vi "Dashboard Main.vi"() -> ()   [LabVIEW 2020]
uses:
  <vilib>/Utility/miscctls.llb/LVRowAndColumnTypeDef.ctl
  <vilib>/event_ctls.llb/eventvkey.ctl
  <vilib>/Rock Robotics/Network Tables/NT Read Numeric Array.vi
  <vilib>/Rock Robotics/WPI/Dashboard/WPI_DashboardLogging Global.vi
panel:
  in  "Camera Settings Right":T1={"Frame Rate"=15, "Compression"=30, "Size"=1, "DB Camera Config"=FALSE} {"Frame Rate" scale=1.0..30.0; "Compression" scale=100.0..-1.0; "Size" items=["640x480", "320x240", "160x120"]}
  in  "Camera Name Right":string(combo)="No Camera Selection"
  out "Camera Perf":string="                          "
  in  "Camera Settings":T1={"Frame Rate"=15, "Compression"=30, "Size"=1, "DB Camera Config"=FALSE} {"Frame Rate" scale=1.0..30.0; "Compression" scale=100.0..-1.0; "Size" items=["640x480", "320x240", "160x120"]}
  in  "TCP":refnum<k5>
  in  "Rec Mode":enum32{"Stop", "Record", "Playback"}(radio)
  out "Robot IP":string="10.11.59.2"
  out "Image Message":string="Timeout in Camera Communications"
  in  "Dashboard Tab":T2(tab)=enum."Custom"
  in  "Select Pickup":string(combo)="Select Pickup ..."
  in  "Select Auto":string(combo)="Select Autonomous ..."
  out "NT Connection":bool
  out "MotorChart R":cluster{"Numeric":dbl, "Numeric":dbl}(graph)
  out "MotorChart L":cluster{"Numeric":dbl, "Numeric":dbl}(graph)
  out "MotorSliders R":cluster{"MotorSlide1":dbl, "MotorSlide2":dbl} {"MotorSlide2" scale=-1.0..1.0 scale format="%#_2e"; "MotorSlide1" scale=-1.0..1.0 scale format="%#_2e"}
  out "MotorSliders L":cluster{"MotorSlide1":dbl, "MotorSlide2":dbl} {"MotorSlide2" scale=-1.0..1.0 scale format="%#_2e"; "MotorSlide1" scale=-1.0..1.0 scale format="%#_2e"}
  out "Gyro":dbl(knob) scale=0.0..360.0
  out "JS1 Z":dbl(slide) scale=-1.0..1.0 scale format="%#_2e"
  out "JS1 Graph":cluster{"X":dbl, "Y":dbl}[](graph)
  out "JS1 Buttons":T3
  out "JS2 Z":dbl(slide) scale=-1.0..1.0 scale format="%#_2e"
  out "JS2 Graph":cluster{"X":dbl, "Y":dbl}[](graph)=[{"X"=0.0, "Y"=-0.007874015748031496}]
  out "JS2 Buttons":T3
  out "Mode":T4(ring)=enum."No Code"
  out "Right Camera Perf":cluster{"Bandwidth (Mbps)":dbl, "FPS":dbl}
  out "Camera Image Right":T5(plugin-control)
  in  "DB/String 9":string
  in  "DB/String 8":string
  in  "DB/String 7":string
  in  "DB/String 6":string
  in  "DB/String 5":string
  in  "DB/String 4":string
  in  "DB/String 3":string
  in  "DB/String 2":string
  in  "DB/String 1":string
  in  "DB/String 0":string
  in  "DB/Slider 0":dbl(slide) scale=0.0..5.0
  in  "DB/Slider 1":dbl(slide) scale=0.0..5.0
  in  "DB/Slider 2":dbl(slide) scale=0.0..5.0
  in  "DB/Slider 3":dbl(slide) scale=0.0..5.0
  out "DB/LED 3":bool
  out "DB/LED 2":bool
  out "DB/LED 1":bool
  out "DB/LED 0":bool
  in  "DB/Button 3":bool
  in  "DB/Button 2":bool
  in  "DB/Button 1":bool
  in  "DB/Button 0":bool caption="New Name"
  in  "Pivot Duration":dbl=1.0
  in  "Pivot Right Speed":dbl=-0.5
  in  "Pivot Left Speed":dbl=0.5
  in  "Transfer Release Duration":dbl=3.0
  in  "Transfer Up Duration":dbl=3.0
  in  "Intake Duration":dbl=5.0
  in  "Shooter Duration":dbl=3.0
  in  "Transfer Release Setpoint":dbl=1.0
  in  "Transfer Up Setpoint":dbl=1.0
  in  "Intake Setpoint":dbl=0.6
  in  "Shooter Setpoint":dbl=1.0
  in  "Test Slider":dbl(slide) scale=0.0..100.0 scale format="%#_3g"
  in  "On/Off":bool caption="Solenoid"
  in  "Test Name":u16(ring) items=["Select the test to run..."]
  in  "Test Tree":string(tree)
  in  "Motor":cluster{"Value":dbl, "Enable":bool} {"Value" scale=-1.0..1.0 scale format="%#_3g"}
  out "Progress":T6 {"Test Progress" scale=0.0..100.0}
  in  "Rev/Fwd":cluster{"Forward":bool, "Reverse":bool}
  in  "Test Ring":u16(ring) items=["Monochrome", "Color"]
  out "Cmd Status":string
  in  "Execute Command":bool
  in  "Command Params":string[][](table)
  in  "Command Selection":i32(listbox)
  in  "CheckList":i32(listbox)
  out "Tree":string(tree)
  out "Camera Image":T5(plugin-control)
  out "Background":bool
  in  "Camera Name":string(combo)="No Camera Selection"
  # "HW"
  # "HW"
  # "Joysticks"
  # "Drive Motors"
  # "Front"
  # "Right"
  # "Left"
  # "Back"
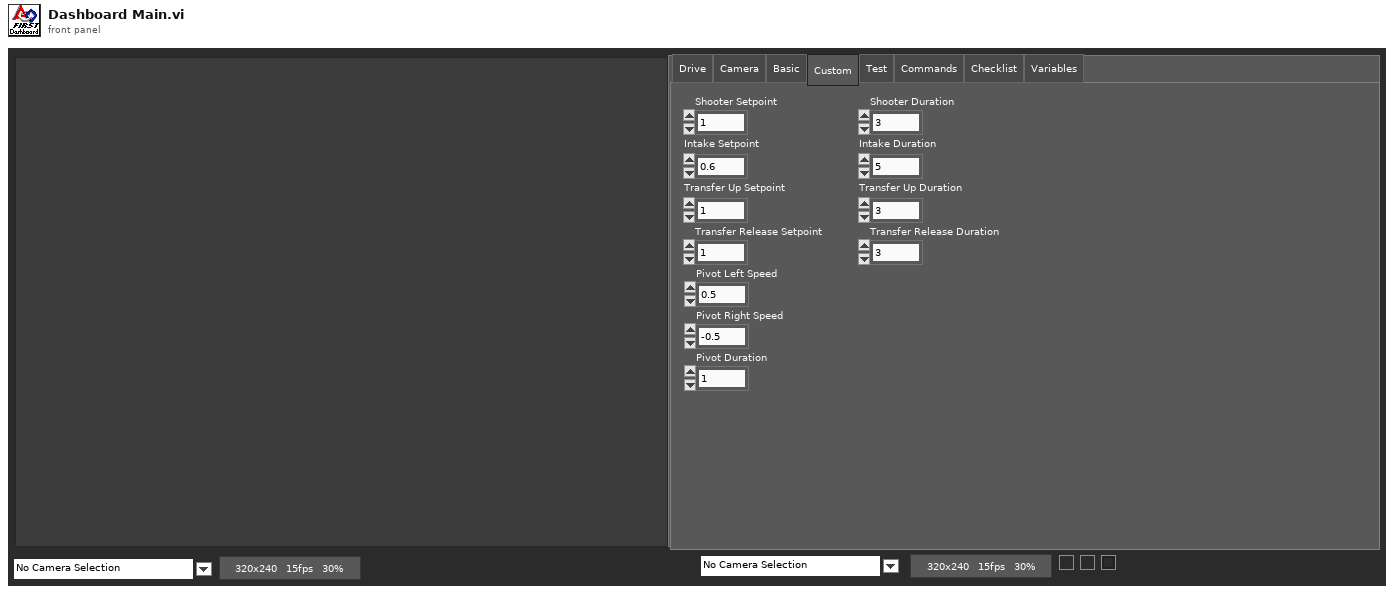
[diagram p1: front panel]
types:
  T1 = cluster{"Frame Rate":i32, "Compression":i32, "Size":u16, "DB Camera Config":bool}
  T2 = enum32{"Drive", "Camera", "Basic", "Custom", "Test", "Commands", "Checklist", "Variables"}
  T3 = cluster{bool, bool, bool, bool, bool, bool, bool, bool, bool, bool, bool, bool}
  T4 = enum8{"Tele-Op Disabled", "Tele-Op Enabled", "Auto Disabled", "Auto Enabled", "Test Disabled", "Test Enabled", "Disconnected", "No Code", "E-Stop"}
  T5 = typedef "IMAQ Image.ctl" = refnum<image>
  T6 = cluster{"Test Progress":u8, "Test Progress Text":string}
  T7 = cluster{"Save Path":path, "Interval (s)":dbl, "Keep":i32}
  T8 = typedef "Image Type" = u32
  T9 = cluster{"IDs":cluster{"RPC field ID":u16, "Unique ID":u16}, "String":string}
  T10 = cluster{"Error Strings":string, "Disable Counts":cluster{u16, u16}, "Rail Faults":cluster{u16, u16, u16}, "Robot IP":string, "DB Mode":u8, "Event Info":cluster{"Name":string, "Type":u8, "Number":u16, "Replay":u8}}
  T11 = cluster{"Storage":cluster{"Disk Free":u64, "RAM Block":u32, "RAM free":u32}, "CPU Utilization":cluster{"CPU % ISR":sgl, "CPU % Time Crit":sgl, "CPU % Timed Str":sgl, "CPU % High":sgl, "CPU % Above":sgl, "CPU % Normal":sgl, "CPU % Low":sgl}, "CAN":cluster{"% Bus Utilization":sgl, "Bus Off Cnt":u32, "TX_FIFO Full Cnt":u32, "Receive Error Cnt":u8, "Transmit Error Cnt":u8}, "HID":cluster{"HID Outputs":u32, "Rumble Low":u16, "Rumble High":u16}[]}
  T12 = cluster{"Status bits":cluster{"Test Mode":bool, "Autonomous":bool, "Enabled":bool, "Code Start":bool, "Brownout":bool, "Reserved 2":bool, "Reserved 3":bool, "E-Stop":bool}, "Code Trace":cluster{"Disabled":bool, "TeleOp":bool, "Auto":bool, "Test":bool}, "Controller Type":enum16{"unknown", "cRIO", "roboRio"}, "Code?":enum16{"unknown", "noCode", "code"}, "Battery V":dbl}
  T13 = cluster{"Control Bits":cluster{"TestMode":bool, "Autonomous":bool, "Enabled":bool, "FMS Present":bool, bool, bool, bool, "E-Stop":bool}, "Team Station ":u8, "Countdown":sgl, "Joystick Values":cluster{"Axes":dbl[], "Buttons":bool[], "POVs":i16[]}[]}
  T14 = cluster{"Axes":dbl[], "Buttons":bool[], "POVs":i16[]}[]
  T15 = cluster{"Axes":dbl[], "Buttons":bool[], "POVs":i16[]}
  T16 = cluster{"Buttons[0]":bool, "Buttons[1]":bool, "Buttons[2]":bool, "Buttons[3]":bool, "Buttons[4]":bool, "Buttons[5]":bool, "Buttons[6]":bool, "Buttons[7]":bool, "Buttons[8]":bool, "Buttons[9]":bool, "Buttons[10]":bool, "Buttons[11]":bool}
  T17 = cluster{"Camera Image":refnum<vi>, "Dashboard Tab":refnum<vi>, "Background":refnum<vi>, "Rec Mode":refnum<vi>, "Test Slider":refnum<vi>, "On/Off ":refnum<vi>, "Test Ring":refnum<vi>, "Rev/Fwd":refnum<vi>, "Test Name":refnum<vi>, "Motor":refnum<vi>, "Progress":refnum<vi>, "CheckList":refnum<vi>, "Tree":refnum<vi>, "Test Tree":refnum<vi>, "Command Params":refnum<vi>, "Command Selection":refnum<vi>, "Execute Command":refnum<vi>, "Cmd Status":refnum<vi>, "Camera Settings":refnum<vi>, "Camera Name":refnum<vi>, "Camera Perf":refnum<vi>, "Camera Settings Right":refnum<vi>, "Camera Name Right":refnum<vi>, "Camera Image Right":refnum<vi>}
  T18 = cluster{"Global Rectangle":i32[], "Contours":cluster{"Contour Type":u32, "ROI Type":u32, "Points":i32[]}[]}
  T19 = cluster{"Camera Name":string, string, "Saved DB Images Info":cluster{"Save Path":path, "Interval (s)":dbl, "Keep":i32}}
  T20 = cluster{"Camera Name Right":string, string, "Saved DB Images Info":cluster{"Save Path":path, "Interval (s)":dbl, "Keep":i32}}
  T21 = cluster{"Operation":enum16{"Update", "Clear"}, "Color Box":u32}[]
  T22 = typedef "eventvkey.ctl" = enum16{"ASCII", "Enter", "Return", "Shift", "Ctrl", "Alt", "Cmd", "Opt", "Caps", "NumLock", "Clear", "Break", "Up", "Down", "Left", "Right", "Insert", "Delete", "Home", "End", "PageUp", "PageDown", "Escape", "Help", "Pause", "ScrollLock", "F1", "F2", "F3", "F4", "F5", "F6", "F7", "F8", "F9", "F10", "F11", "F12", "F13", "F14", "F15", "F16", "F17", "F18", "F19", "F20", "F21", "F22", "F23", "F24", "Play", "VolumeUp", "VolumeDown", "Mute", "Two Byte Char"}
  T23 = cluster{"Image Size":bool, "Image Type":bool, "Pixel Value":bool, "ROI Information":bool, "Zoom Factor":bool}
  T24 = cluster{"Operation":enum16{"Update", "Clear"}, "Color Box":u32}
  T25 = typedef "LVRowAndColumnTypeDef.ctl" = cluster{"Row":i32, "Column":i32}
  T26 = cluster{"Shift":bool, "Ctrl":bool, "Alt":bool, "Cmd":bool, "Opt":bool}
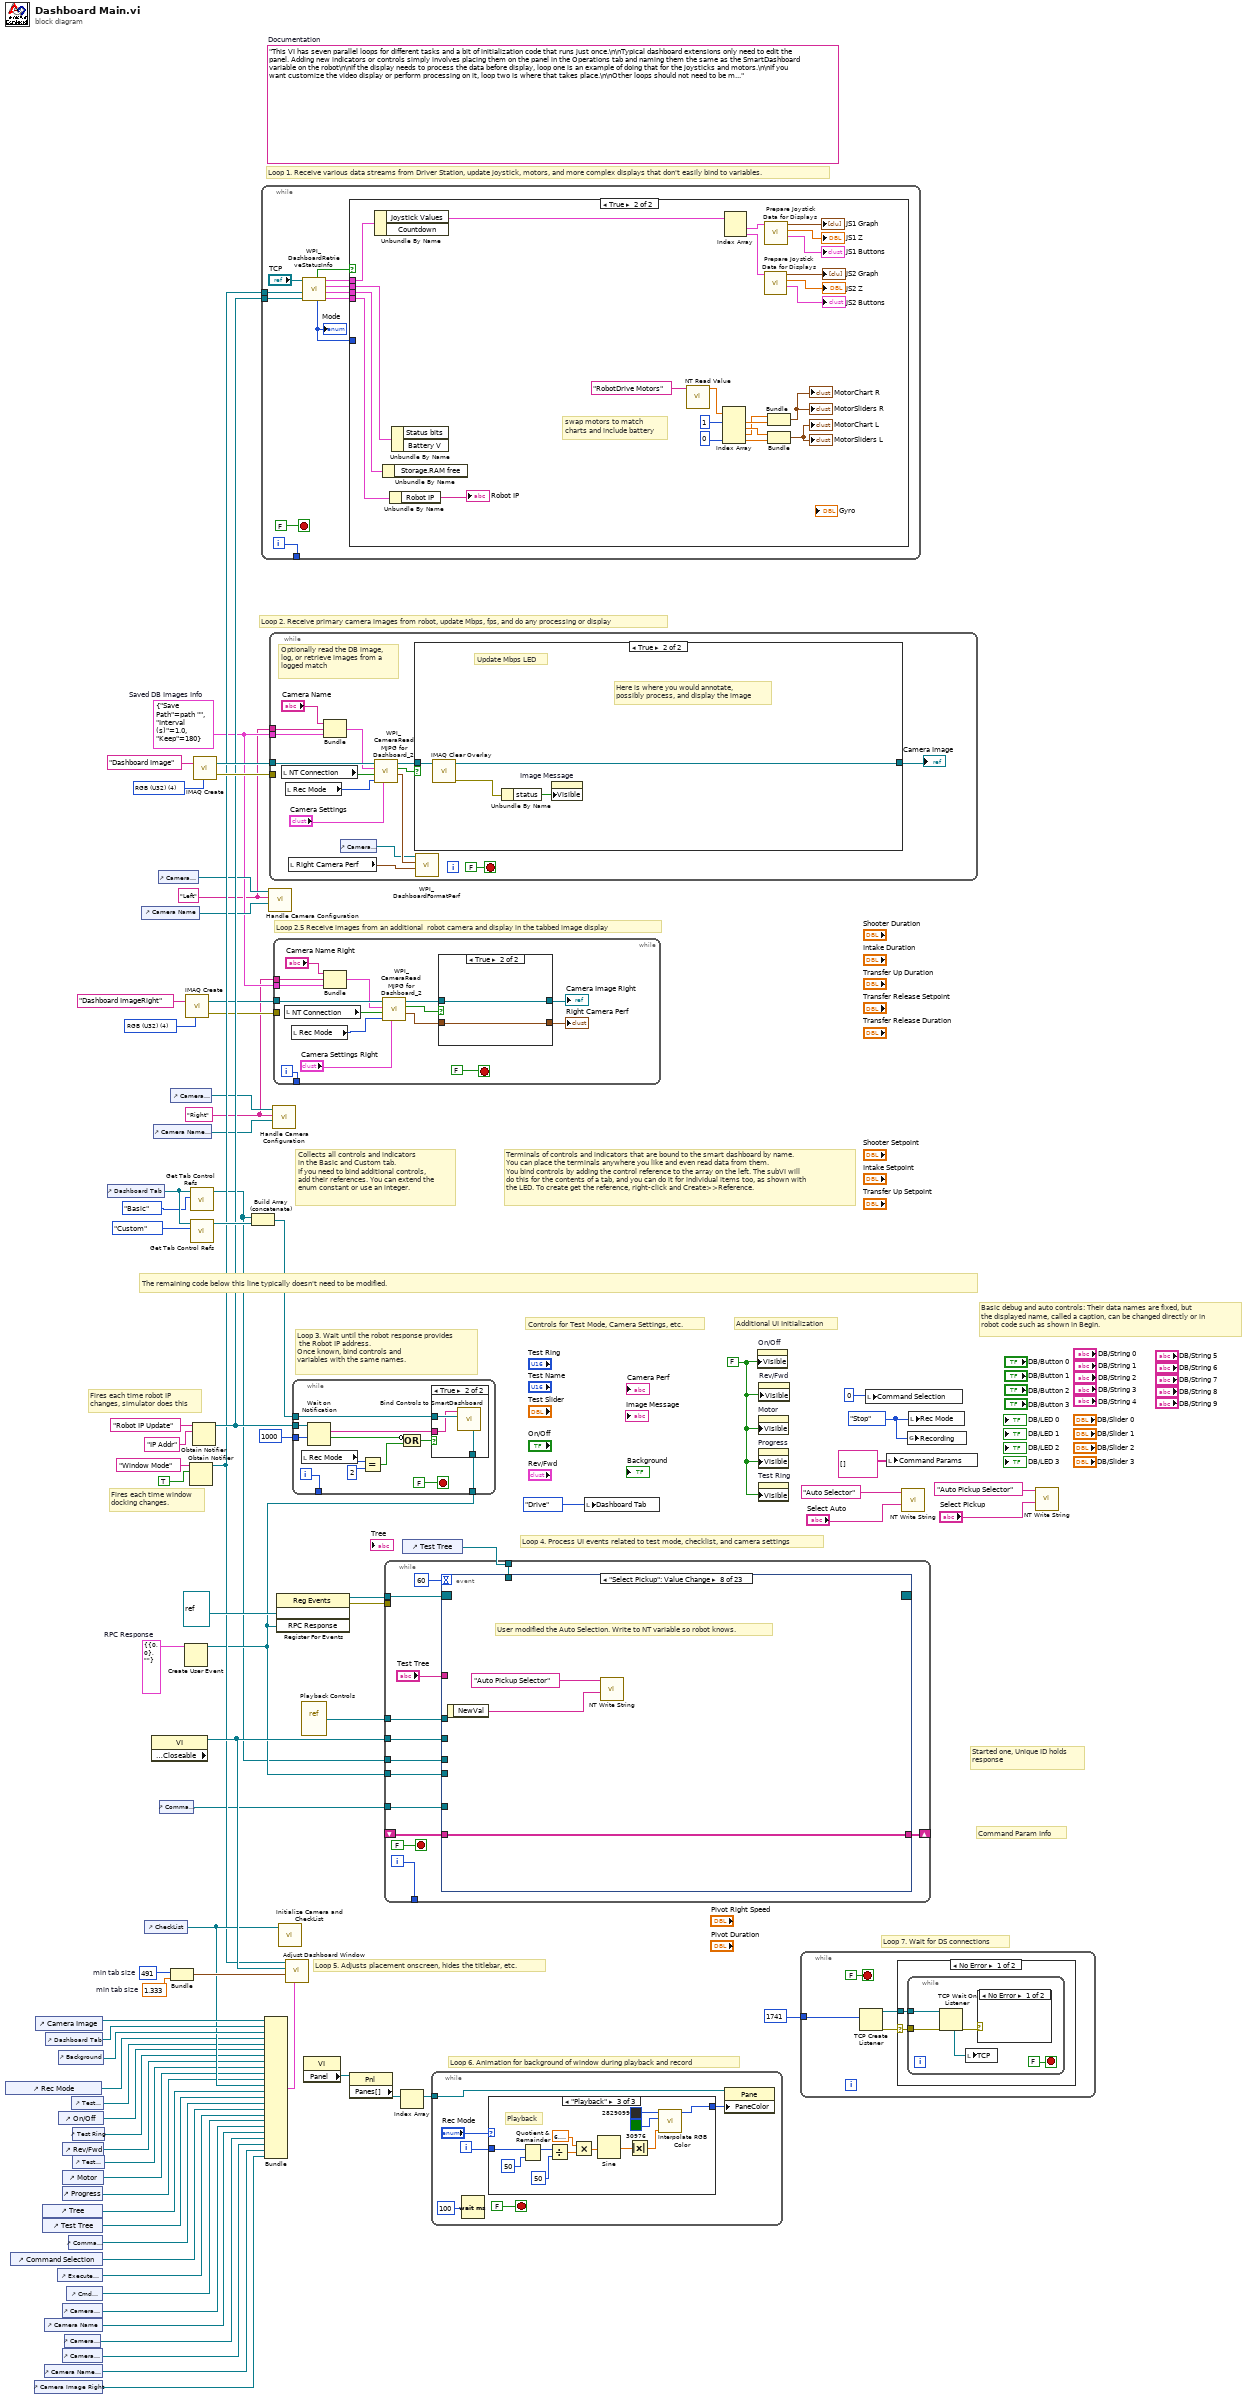
[diagram p0: block diagram]
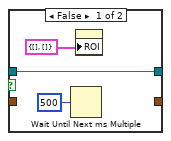
[diagram p2: hidden frame]
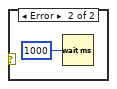
[diagram p3: hidden frame]
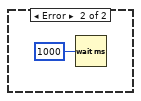
[diagram p4: hidden frame]
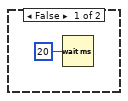
[diagram p5: hidden frame]
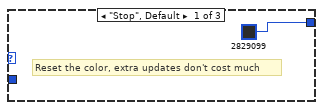
[diagram p6: hidden frame]
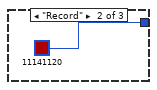
[diagram p7: hidden frame]
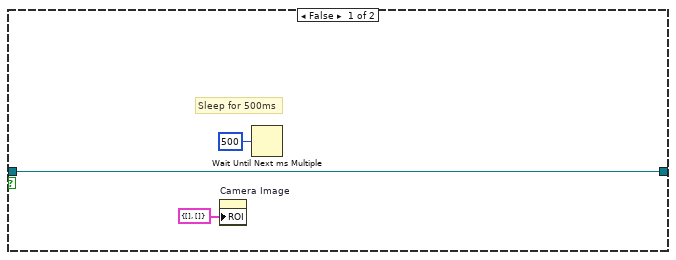
[diagram p9: hidden frame]
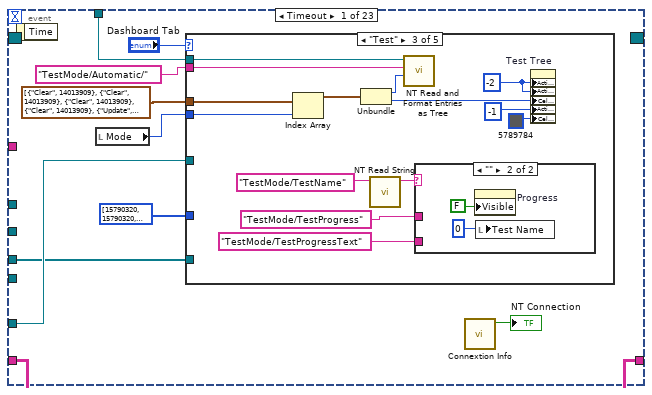
[diagram p10: hidden frame]
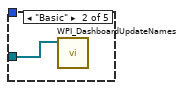
[diagram p12: hidden frame]
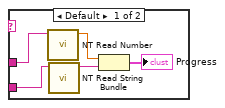
[diagram p13: hidden frame]
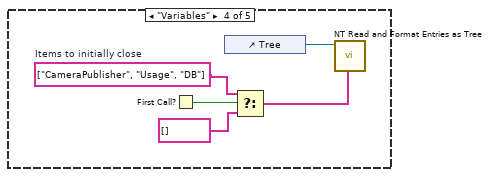
[diagram p14: hidden frame]
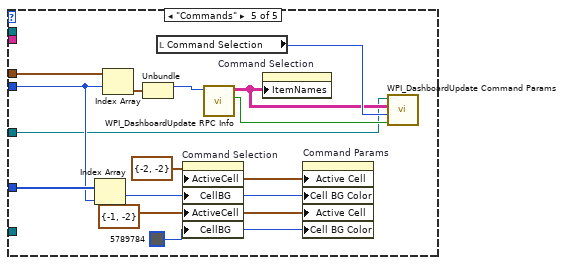
[diagram p15: hidden frame]
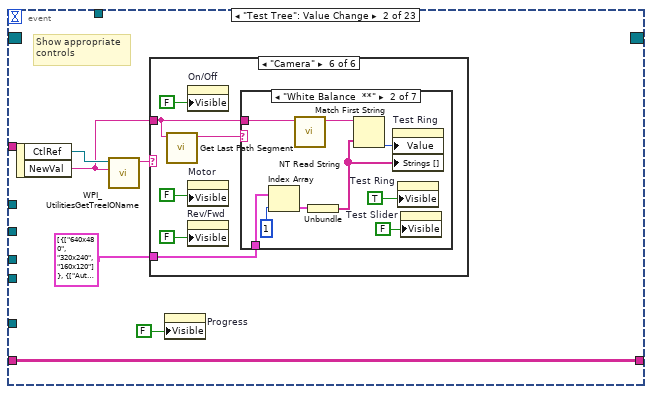
[diagram p16: hidden frame]
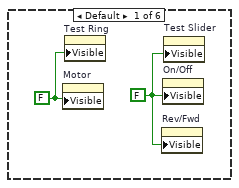
[diagram p17: hidden frame]
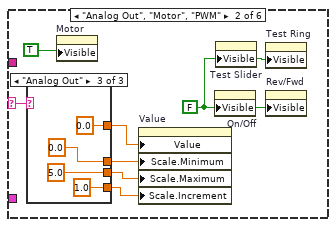
[diagram p18: hidden frame]
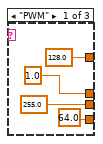
[diagram p19: hidden frame]
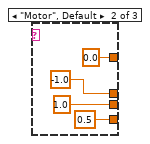
[diagram p20: hidden frame]
diagram:
  w5 = T7 {"Save Path"=path "", "Interval (s)"=1.0, "Keep"=180}  # Saved DB Images Info
  w4 = "Right"
  w3 = "Left"
  w15 = T8 4 items=["Grayscale (U8)", "Grayscale (I16)", "Grayscale (SGL)", "Complex (CSG)", "RGB (U32)", "HSL (U32)", "RGB (U64)"] ("Image Type")
  w31 = T9 {"IDs"={"RPC field ID"=0, "Unique ID"=0}, "String"=""}  # RPC Response
  w54 = 491  # min tab size
  w53 = 1.333  # min tab size
  w61 = enum32{"Stop", "Record", "Playback"}."Stop" ("Rec Mode")
  w38 = FALSE ("Visible")
  (unwired) "This VI has seven parallel loops for different tasks and a bit of initialization code that runs just once.\n\nTypical dashboard extensions only need to edit the panel. Adding new indicators or controls simply involves placing them on the panel in the Operations tab and naming them the same as the SmartDashboard variable on the robot\n\nIf the display needs to process the data before display, loop one is an example of doing that for the joysticks and motors.\n\nIf you want customize the video display or perform processing on it, loop two is where that takes place.\n\nOther loops should not need to be modified. They are pretty standard, and document the task they perform."  # Documentation
  w78 = T8 4 items=["Grayscale (U8)", "Grayscale (I16)", "Grayscale (SGL)", "Complex (CSG)", "RGB (U32)", "HSL (U32)", "RGB (U64)"] ("Image Type")
  # "Loop 2.5 Receive images from an additional  robot camera and display in the tabbed image display"
  # "Command Param Info"
  # "Started one, Unique ID holds\nresponse"
  # "Loop 7. Wait for DS connections"
  # "Basic debug and auto controls: Their data names are fixed, but\nthe displayed name, called a caption, can be changed directly or in\nrobot code such as shown in Begin."
  # "Controls for Test Mode, Camera Settings, etc."
  # "Additional UI Initialization"
  # "Loop 6. Animation for background of window during playback and record"
  # "Fires each time robot IP\nchanges, simulator does this"
  # "Fires each time window\ndocking changes."
  # "Collects all controls and indicators\nin the Basic and Custom tab.\nIf you need to bind additional controls,\nadd their references. You can extend the\nenum constant or use an integer."
  # "The remaining code below this line typically doesn't need to be modified."
  # "Loop 4. Process UI events related to test mode, checklist, and camera settings"
  # "Terminals of controls and indicators that are bound to the smart dashboard by name.\nYou can place the terminals anywhere you like and even read data from them.\nYou bind controls by adding the control reference to the array on the left. The subVI will\ndo this for the contents of a tab, and you can do it for individual items too, as shown with\nthe LED. To create get the reference, right-click and Create>>Reference."
  # "Loop 3. Wait until the robot response provides\n the Robot IP address.\nOnce known, bind controls and\nvariables with the same names."
  # "Loop 5. Adjusts placement onscreen, hides the titlebar, etc."
  # "Loop 1. Receive various data streams from Driver Station, update joystick, motors, and more complex displays that don't easily bind to variables."
  # "Loop 2. Receive primary camera images from robot, update Mbps, fps, and do any processing or display"
  n1 = control-ref of="Rec Mode"() -> (w44:refnum<vi>)
  n2 = control-ref of="Command Selection"() -> (w30:refnum<vi>)
  n3 = control-ref of="Camera Image Right"() -> (w8:refnum<vi>)
  n4 = control-ref of="Camera Image"() -> (w56:refnum<vi>)
  n5 = control-ref of="Tree"() -> (w48:refnum<vi>)
  n6 = control-ref of="Test Tree"() -> (w47:refnum<vi>)
  n7 = control-ref of="Camera Name"() -> (w21:refnum<vi>)
  n8 = control-ref of="Camera Name Right"() -> (w9:refnum<vi>)
  n9 = control-ref of="Dashboard Tab"() -> (w55:refnum<vi>)
  n10 = control-ref of="Execute Command"() -> (w32:refnum<vi>)
  n11 = control-ref of="Background"() -> (w51:refnum<vi>)
  n12 = control-ref of="On/Off"() -> (w42:refnum<vi>)
  n13 = control-ref of="Progress"() -> (w39:refnum<vi>)
  n14 = control-ref of="Camera Settings"() -> (w22:refnum<vi>)
  n15 = control-ref of="Camera Settings Right"() -> (w10:refnum<vi>)
  n16 = control-ref of="Rev/Fwd"() -> (w40:refnum<vi>)
  n17 = control-ref of="Motor"() -> (w45:refnum<vi>)
  n18 = control-ref of="Camera Perf"() -> (w20:refnum<vi>)
  n19 = control-ref of="Cmd Status"() -> (w26:refnum<vi>)
  n20 = control-ref of="Command Params"() -> (w33:refnum<vi>)
  n21 = control-ref of="Test Slider"() -> (w43:refnum<vi>)
  n22 = control-ref of="Test Ring"() -> (w41:refnum<vi>)
  n23 = control-ref of="Test Name"() -> (w46:refnum<vi>)
  n24 = control-ref of="Dashboard Tab"() -> (w59:refnum<vi>)
  n25 = control-ref of="Camera Name"() -> (w23:refnum<vi>)
  n26 = control-ref of="CheckList"() -> (w49:refnum<vi>)
  n27 = property class="VI" props=["Front Panel.Closeable"]() -> (reference out=w60:refnum<vi>)  [unwired: 2 in, 2 out]
  n28 = control-ref of="Camera Name Right"() -> (w11:refnum<vi>)
  n29 = control-ref of="Camera Settings"() -> (w24:refnum<vi>)
  n30 = control-ref of="Command Params"() -> (w25:refnum<vi>)
  n31 = control-ref of="Camera Settings Right"() -> (w12:refnum<vi>)
  n32 = Bundle("min tab size"=w54, "min tab size"=w53) -> (w52:cluster{"min tab size":i32, "min tab size":dbl})  [unwired: 1 in]
  n33 = Create User Event(user event datatype=w31) -> (user event=w27:refnum<user-event>)  [unwired: 1 in, 1 out]
  n34 = call "IMAQ Create"("Image Name"="Dashboard ImageRight", "Image Type"=w15) -> ("New Image"=w14:T5, "error out"=w13:errorcluster)  [unwired: 2 in, 1 out]
  n35 = Obtain Notifier(name (unnamed)="Window Mode", notification data type=TRUE) -> (notifier out=w36:refnum<notifier>)  [unwired: 2 in, 2 out]
  n36 = call <vilib>:"Get Tab Control Refs.vi"("Page Index"=T2."Basic" ("Dashboard Tab"), "TabControl in"=w59) -> ("ControlsOnPage"=w19:refnum<vi>[])  [unwired: 9 in]
  n37 = call <vilib>:"Get Tab Control Refs.vi"("Page Index"=T2."Custom" ("Dashboard Tab"), "TabControl in"=w59) -> ("ControlsOnPage"=w58:refnum<vi>[])  [unwired: 9 in]
  n38 = Obtain Notifier(name (unnamed)="Robot IP Update", notification data type="IP Addr" ("name (unnamed)")) -> (notifier out=w37:refnum<notifier>)  [unwired: 2 in, 2 out]
  n39 = call "IMAQ Create"("Image Name"="Dashboard Image", "Image Type"=w78) -> ("New Image"=w76:T5, "error out"=w75:errorcluster)  [unwired: 2 in, 1 out]
  n40 = Build Array (concatenate)(w19, w58) -> (w57:refnum<vi>[])
  n41 = while {
    tunnel: [w88] -> _
    tunnel: w37 -> [w82]
    tunnel: w36 -> [w79]
    i -> [w88]
    stop <- FALSE stop-if-true
    n42 = call <vilib>:"WPI_DashboardRetrieveStatusInfo.vi"("Binding Refnum"=w82, "Window Mode Notifier"=w79, "TCP Cnx"="TCP") -> ("Power and Errors"=w83:T10, "Robot Metrics"=w86:T11, "Status Info"=w87:T12, "Control Info"=w84:T13, "Robot Mode"=w81:T4, "Process?"=w85:bool)  [unwired: 3 in]
    "Mode" <- w81
    n43 = case shown="True" w85 {
      tunnel: w87 -> [_ w114]
      tunnel: w86 -> [_ w113]
      tunnel: w84 -> [_ w112]
      tunnel: w83 -> [_ w111]
      tunnel: w81 -> [_ _]
      frame False {
        n44 = Wait (ms)(milliseconds to wait=u32 20) -> ()  [unwired: 1 out]
      }
      frame True {
        # "swap motors to match\ncharts and include battery"
        n45 = Unbundle By Name(w112) -> ("Joystick Values"=w102:T14)  [unwired: 1 out]
        n46 = Unbundle By Name(w113) -> ()  [unwired: 1 out]
        n47 = Unbundle By Name(w111) -> ("Robot IP"=→"Robot IP":string)
        n48 = Unbundle By Name(w114) -> ()  [unwired: 2 out]
        n49 = call-poly <vilib>:"NT Read Value.vi"("Name"="RobotDrive Motors") -> ("Numeric Array"=w92:dbl[])  [unwired: 9 in, 1 out]
        n50 = Index Array(array=w92, index #1=1, index #4=0) -> (element #1=w106:dbl, element #2=w107:dbl, element #3=w105:dbl, element #4=w110:dbl)  [unwired: 2 in]
        n51 = Index Array(array=w102) -> (element #1=w101:T15, element #2=w97:T15)  [unwired: 2 in]
        n52 = call "Prepare Joystick Data for Displays.vi"("Joystick Values"=w97) -> ("Buttons"=→"JS2 Buttons":T16, "Z Axis"=→"JS2 Z":dbl, "Cartesian Data"=→"JS2 Graph":cluster{"X axis":dbl, "X axis":dbl}[])  [unwired: 8 in]
        n53 = call "Prepare Joystick Data for Displays.vi"("Joystick Values"=w101) -> ("Buttons"=→"JS1 Buttons":T16, "Z Axis"=→"JS1 Z":dbl, "Cartesian Data"=→"JS1 Graph":cluster{"X axis":dbl, "X axis":dbl}[])  [unwired: 8 in]
        n54 = Bundle("Numeric"=w105, "Numeric"=w106) -> (→"MotorChart R" →"MotorSliders R":cluster{"Numeric":dbl, "Numeric":dbl})  [unwired: 1 in]
        n55 = Bundle("Numeric"=w107, "Numeric"=w110) -> (→"MotorChart L" →"MotorSliders L":cluster{"Numeric":dbl, "Numeric":dbl})  [unwired: 1 in]
      }
    }
  }
  n56 = Bundle("Camera Image"=w56, "Dashboard Tab"=w55, "Background"=w51, "Rec Mode"=w44, "Test Slider"=w43, "On/Off"=w42, "Test Ring"=w41, "Rev/Fwd"=w40, "Test Name"=w46, "Motor"=w45, "Progress"=w39, "CheckList"=w49, "Tree"=w48, "Test Tree"=w47, "Command Params"=w33, "Command Selection"=w30, "Execute Command"=w32, "Cmd Status"=w26, "Camera Settings"=w22, "Camera Name"=w21, "Camera Perf"=w20, "Camera Settings Right"=w10, "Camera Name Right"=w9, "Camera Image Right"=w8) -> (w50:T17)  [unwired: 1 in]
  n57 = call "Handle Camera Configuration.vi"("CameraNameRef"=w23, "Display Name"=w3, "ClusterRef"=w24) -> ()  [unwired: 9 in]
  n58 = while {
    tunnel: w76 -> [w128]
    tunnel: w75 -> [_]
    tunnel: w5 -> [w121]
    tunnel: w3 -> [w118]
    stop <- FALSE stop-if-true
    # "Optionally read the DB image,\nlog, or retrieve images from a\nlogged match"
    n59 = local read "NT Connection"() -> (w122:bool)
    n60 = local read "Rec Mode"() -> (w125:enum32{"Stop", "Record", "Playback"})
    n61 = local read "Right Camera Perf"() -> (w116:cluster{"Bandwidth (Mbps)":dbl, "FPS":dbl})
    n62 = Bundle("Camera Name"="Camera Name", w118, "Saved DB Images Info"=w121) -> (w120:T19)  [unwired: 1 in]
    n63 = control-ref of="Camera Perf"() -> (w115:refnum<vi>)
    n64 = call <vilib>:"WPI_CameraRead MJPG for Dashboard_2.vi"("Camera Settings"="Camera Settings", "Rec Mode"=w125, "NT Connection"=w122, "Capture Info"=w120, "Image in"=w128) -> ("perf info"=w117:cluster{"Bandwidth (Mbps)":dbl, "fps":dbl}, "Active"=w126:bool, "Image\\ out"=w127:T5)  [unwired: 4 in]
    n65 = case shown="True" w126 {
      tunnel: w127 -> [w131 w134]
      tunnel: [w131 w133] -> w123
      frame False {
        # "Sleep for 500ms"
        n66 = property on="Camera Image" class="ImageControl"("ROI"=T18 {"Global Rectangle"=[], "Contours"=[]}) -> ()  [unwired: 2 in, 2 out]
        n67 = Wait Until Next ms Multiple(millisecond multiple=u32 500) -> ()  [unwired: 1 out]
      }
      frame True {
        # "Here is where you would annotate,\npossibly process, and display the image"
        # "Update Mbps LED"
        n68 = call "IMAQ Clear Overlay"("Image"=w134) -> ("error out"=w135:errorcluster, "Image Out"=w133:T5)  [unwired: 2 in, 7 out]
        n69 = Unbundle By Name(w135) -> ("status"=w136:bool)
        n70 = property on="Image Message" class="Str"("Visible"=w136) -> ()  [unwired: 2 in, 2 out]
      }
    }
    "Camera Image" <- w123
    n71 = call <vilib>:"WPI_DashboardFormatPerf.vi"("Right Camera Perf"=w116, "Performance"=w117, "String in"=w115) -> ()  [unwired: 9 in]
  }
  n72 = call "Handle Camera Configuration.vi"("CameraNameRef"=w11, "Display Name"=w4, "ClusterRef"=w12) -> ()  [unwired: 9 in]
  n73 = while {
    tunnel: w14 -> [w151]
    tunnel: w13 -> [_]
    tunnel: [w146] -> _
    tunnel: w5 -> [w142]
    tunnel: w4 -> [w139]
    i -> [w146]
    stop <- FALSE stop-if-true
    n74 = local read "NT Connection"() -> (w143:bool)
    n75 = local read "Rec Mode"() -> (w150:enum32{"Stop", "Record", "Playback"})
    n76 = Bundle("Camera Name Right"="Camera Name Right", w139, "Saved DB Images Info"=w142) -> (w141:T20)  [unwired: 1 in]
    n77 = call <vilib>:"WPI_CameraRead MJPG for Dashboard_2.vi"("Camera Settings"="Camera Settings Right", "Rec Mode"=w150, "NT Connection"=w143, "Capture Info"=w141, "Image in"=w151) -> ("perf info"=w137:cluster{"Bandwidth (Mbps)":dbl, "fps":dbl}, "Active"=w145:bool, "Image\\ out"=w148:T5)  [unwired: 4 in]
    n78 = case shown="True" w145 {
      tunnel: w148 -> [w153 w156]
      tunnel: [w153 w156] -> w144
      tunnel: [_ w155] -> w138
      tunnel: w137 -> [_ w155]
      frame False {
        n79 = Wait Until Next ms Multiple(millisecond multiple=u32 500) -> ()  [unwired: 1 out]
        n80 = property on="Camera Image Right" class="ImageControl"("ROI"=T18 {"Global Rectangle"=[], "Contours"=[]}) -> ()  [unwired: 2 in, 2 out]
      }
      frame True {
      }
    }
    "Camera Image Right" <- w144
    "Right Camera Perf" <- w138
  }
  n81 = register-events(refnum<vi> refnum, w27) -> (reference out=w65:refnum<event-registration>, error out=w64:errorcluster)  [unwired: 2 in]
  n82 = call "Initialize Camera and CheckList.vi"("ListBox in"=w49) -> ()  [unwired: 11 in]
  n83 = call "Adjust Dashboard Window.vi"("Sizing Refnums"=w50, "Size Constraints"=w52, "VI"=w60, "WIn Mode"=w36) -> ()  [unwired: 8 in]
  n84 = while {
    tunnel: w57 -> [w168]
    tunnel: w37 -> [w166]
    tunnel: [w164] -> _
    tunnel: u32 1000 ("milliseconds to wait") -> [w163]
    tunnel: w27 -> [w157]
    i -> [w164]
    stop <- FALSE stop-if-true
    n85 = local read "Rec Mode"() -> (w159:enum32{"Stop", "Record", "Playback"})
    n86 = Wait on Notification(notifier=w166, timeout in ms (-1)=w163) -> (notification=w165:string, timed out?=w161:bool)  [unwired: 2 in, 2 out]
    n87 = Equal?(x=w159, y=u16 2 ("Rec Mode")) -> (x = y?=w160:bool)
    n88 = Compound Arithmetic op=OR(invert w161, w160) -> (w162:bool)
    n89 = case shown="True" w162 {
      tunnel: w168 -> [_ w171]
      tunnel: w165 -> [_ w170]
      tunnel: w157 -> [_ w169]
      frame False {
      }
      frame True {
        n90 = call <vilib>:"Bind Controls to SmartDashboard.vi"("RPC ref"=w169, "Bound Control Refs"=w171, "Server IP Address"=w170) -> ()  [unwired: 9 in]
      }
    }
  }
  n91 = vi-ref "Playback Controls.vi"() -> (w66:refnum<vi>)
  n92 = property class="VI"() -> ("Panel"=w68:refnum<vi>)  [unwired: 2 in, 2 out]
  n93 = property class="Pnl"(reference=w68) -> ("Panes[]"=w69:refnum<vi>[])  [unwired: 1 in, 2 out]
  n94 = Index Array(array=w69) -> (element=w67:refnum<vi>)  [unwired: 1 in]
  n95 = control-ref of="Test Tree"() -> (w70:refnum<vi>)
  n96 = while {
    tunnel: [w181] -> _
    tunnel: w70 -> [w180]
    tunnel: w66 -> [w179]
    tunnel: w65 -> [w178]
    tunnel: w64 -> [_]
    tunnel: w60 -> [w177]
    tunnel: w27 -> [w176]
    tunnel: w25 -> [w175]
    shift-right: [w174] -> _
    shift-left: _ -> [w173]
    tunnel: w19 -> [w172]
    i -> [w181]
    stop <- FALSE stop-if-true
    n97 = event shown="[7] \"Select Pickup\": Value Change" {
      selector: w178 -> [_ _ _ _ _ _ _ _ _ _ _ _ _ _ _ _ _ _ _ _ _ _ _]
      dyn-events: [_ _ _ _ _ _ _ _ _ _ _ _ _ _ _ _ _ _ w447 _ _ _ _] -> _
      timeout: u32 60 ("milliseconds to wait") -> [_ _ _ _ _ _ _ _ _ _ _ _ _ _ _ _ _ _ _ _ _ _ _]
      tunnel: w180 -> [w193 _ _ _ _ _ _ _ _ _ _ _ _ _ _ _ _ _ _ _ _ _ _]
      tunnel: "Test Tree" -> [_ _ _ _ _ _ _ _ _ _ _ _ _ w414 w422 w424 w428 w436 _ _ _ _ _]
      tunnel: w179 -> [_ _ _ _ _ _ _ _ _ _ _ _ _ _ _ _ _ _ w449 _ w467 _ _]
      tunnel: w177 -> [_ _ _ _ _ _ _ _ _ _ _ _ _ _ _ _ _ _ w445 _ _ _ _]
      tunnel: w176 -> [_ _ _ _ _ _ _ _ _ _ _ _ _ _ _ _ _ _ w443 _ _ _ _]
      tunnel: w175 -> [w188 _ _ _ _ _ _ _ w365 _ _ _ _ _ _ _ _ _ _ _ _ _ _]
      tunnel: [w187 w236 w338 w343 w352 w356 w359 w362 w363 w372 w382 w389 w401 w413 w420 w423 w427 w435 w442 w462 w464 w468 w481] -> w174
      tunnel: w173 -> [w187 w236 w338 w343 w352 w356 w359 w362 w363 _ _ w389 w401 w413 w420 w423 w427 w435 w442 w462 w464 w468 w481]
      tunnel: w172 -> [w185 _ _ _ _ _ _ _ _ _ _ _ _ _ _ _ _ _ _ _ _ _ _]
      event Timeout {
        n98 = event-data() -> ()  [unwired: 1 in, 1 out]
        n99 = local read "Mode"() -> (w190:T4)
        n100 = case shown="\"Test\"" "Dashboard Tab" {
          tunnel: w193 -> [_ _ w209 _ _]
          tunnel: "TestMode/Automatic/" ("Name Pattern") -> [_ _ w208 _ _]
          tunnel: T21 [{"Operation"=enum."Clear", "Color Box"=14013909}, {"Operation"=enum."Clear", "Color Box"=14013909}, {"Operation"=enum."Clear", "Color Box"=14013909}, {"Operation"=enum."Clear", "Color Box"=14013909}, {"Operation"=enum."Update", "Color Box"=14013909}, {"Operation"=enum."Update", "Color Box"=16777215}, {"Operation"=enum."Clear", "Color Box"=14013909}, {"Operation"=enum."Clear", "Color Box"=14013909}, {"Operation"=enum."Clear", "Color Box"=14013909}] -> [_ _ w201 _ w229]
          tunnel: w190 -> [_ _ w200 _ w228]
          tunnel: u32[] [15790320, 15790320, 15790320, 15790320, 16777215, 16777215, 15790320, 15790320, 15790320] -> [_ _ _ _ w234]
          tunnel: w188 -> [_ _ _ _ w222]
          tunnel: w185 -> [_ w195 _ _ _]
          frame "Custom", Default {
          }
          frame "Basic" {
            n101 = call <vilib>:"WPI_DashboardUpdateNames.vi"("Controls on Tab"=w195) -> ()  [unwired: 11 in]
          }
          frame "Test" {
            w207 = -2 ("Active Item:Row Number")
            n102 = Index Array(array=w201, index=w200) -> (element=w202:T24)
            n103 = Unbundle(w202) -> ("Operation"=w203:enum16{"Update", "Clear"}, "Color Box"=w204:u32)
            n104 = call <vilib>:"NT Read String.vi"("Name"="TestMode/TestName") -> ("String"=w198:string)  [unwired: 9 in, 1 out]
            n105 = call <vilib>:"NT Read and Format Entries as Tree.vi"("Operation"=w203, "Name Pattern"=w208, "Tree Refnum"=w209) -> ()  [unwired: 7 in, 2 out]
            n106 = case shown="\"\"" w198 {
              tunnel: "TestMode/TestProgress" ("Name") -> [w211 _]
              tunnel: "TestMode/TestProgressText" ("Name") -> [w210 _]
              frame Default {
                n107 = call <vilib>:"NT Read Number.vi"("Name"=w211) -> ("Numeric"=w212:dbl)  [unwired: 9 in, 1 out]
                n108 = call <vilib>:"NT Read String.vi"("Name"=w210) -> ("String"=w213:string)  [unwired: 9 in, 1 out]
                n109 = Bundle("Numeric"=w212, "String"=w213) -> (→"Progress":cluster{"Numeric":dbl, "String":string})  [unwired: 1 in]
              }
              frame "" {
                n110 = property on="Progress" class="Clust (strict)"("Visible"=FALSE) -> ()  [unwired: 2 in, 2 out]
                n111 = local write "Test Name"(u16 0) -> ()
              }
            }
            n112 = property on="Test Tree" class="Tree (strict)"("Active Item Row Number"=w207, "ActiveColNum"=w207, "CellBG"=w204, "Active Item Row Number"=-1 ("Active Item:Row Number"), "CellBG"=u32 5789784 ("Color Box")) -> ()  [unwired: 2 in, 2 out]
          }
          frame "Variables" {
            w219 = string[] ["CameraPublisher", "Usage", "DB"]  # Items to initially close
            n113 = First Call?() -> (First Call?: T/F=w220:bool)
            n114 = control-ref of="Tree"() -> (w221:refnum<vi>)
            n115 = Select(t=w219, s=w220, f=string[] []) -> (s? t:f=w217:string[])
            n116 = call <vilib>:"NT Read and Format Entries as Tree.vi"("Tags to  Close"=w217, "Tree Refnum"=w221) -> ()  [unwired: 8 in, 2 out]
          }
          frame "Commands" {
            w230 = u32 5789784 ("Color Box")
            w231 = T25 {"Row"=-1, "Column"=-2} ("Active Cell:Active Cell")
            w233 = T25 {"Row"=-2, "Column"=-2} ("Active Cell:Active Cell")
            n117 = Index Array(array=w234, index=w228) -> (element=w232:u32)
            n118 = Index Array(array=w229, index=w228) -> (element=w227:T24)
            n119 = Unbundle(w227) -> ("Operation"=w226:enum16{"Update", "Clear"})  [unwired: 1 out]
            n120 = local read "Command Selection"() -> (w225:i32)
            n121 = property on="Command Selection" class="MCListbox (strict)"("ActiveCell"=w233, "CellBG"=w232, "ActiveCell"=w231, "CellBG"=w230) -> ()  [unwired: 2 in, 2 out]
            n122 = call <vilib>:"WPI_DashboardUpdate RPC Info.vi"("Operation"=w226) -> ("update"=w224:bool, "commands"=w223:string[][])  [unwired: 9 in]
            n123 = property on="Command Selection" class="MCListbox (strict)"("ItemNames"=w223) -> ()  [unwired: 2 in, 2 out]
            n124 = property on="Command Params" class="Tbl (strict)"("Active Cell"=w233, "Cell BG Color"=w232, "Active Cell"=w231, "Cell BG Color"=w230) -> ()  [unwired: 2 in, 2 out]
            n125 = call <vilib>:"WPI_DashboardUpdate Command Params.vi"("Update"=w224, "NewVal"=w225, "Commands"=w223, "Param Tbl"=w222) -> ()  [unwired: 7 in, 1 out]
          }
        }
        n126 = call <vilib>:"Connextion Info.vi"() -> ("Connected"=→"NT Connection":bool)  [unwired: 10 in, 1 out]
      }
      event "Test Tree": Value Change {
        # "Show appropriate\ncontrols"
        n127 = event-data() -> ("CtlRef"=w239:refnum<vi>, "NewVal"=w237:string)  [unwired: 1 in]
        n128 = call <vilib>:"WPI_UtilitiesGetTreeIOName.vi"("NewVal"=w237, "TreeControl in"=w239) -> ("I/O Name"=w240:string)  [unwired: 9 in]
        n129 = case shown="\"Camera\"" w240 {
          selector: w240 -> [_ w247 _ w269 w278 _]
          tunnel: w237 -> [_ _ w266 w268 _ w285]
          tunnel: cluster{string[]}[] [{["640x480", "320x240", "160x120"]}, {["Auto", "Fixed indoor", "Fixed outdoor 1", "Fixed outdoor 2", "Fixed fluorescent 1", "Fixed fluorescent 2", "Hold current"]}, {["Auto", "Flicker-free 50 Hz", "Flicker-free 60 Hz", "Hold current"]}, {["None", "Prioritize frame rate", "Prioritize image quality"]}, {["Monochrome", "Color"]}] -> [_ _ _ _ _ w284]
          frame Default {
            w242 = FALSE ("Visible")
            w241 = FALSE ("Visible")
            n130 = property on="Motor" class="Clust (strict)"("Visible"=w241) -> ()  [unwired: 2 in, 2 out]
            n131 = property on="Test Ring" class="Ring (strict)"("Visible"=w241) -> ()  [unwired: 2 in, 2 out]
            n132 = property on="Rev/Fwd" class="Clust (strict)"("Visible"=w242) -> ()  [unwired: 2 in, 2 out]
            n133 = property on="On/Off" class="Bool (strict)"("Visible"=w242) -> ()  [unwired: 2 in, 2 out]
            n134 = property on="Test Slider" class="Slide (strict)"("Visible"=w242) -> ()  [unwired: 2 in, 2 out]
          }
          frame "Analog Out", "Motor", "PWM" {
            w248 = FALSE ("Visible")
            n135 = case shown="\"Analog Out\"" w247 {
              tunnel: [1.0 ("Value") -1.0 ("Value") 0.0 ("Value")] -> w246
              tunnel: [255.0 ("Value") 1.0 ("Value") 5.0 ("Value")] -> w245
              tunnel: [128.0 ("Value") 0.0 ("Value") 0.0 ("Value")] -> w244
              tunnel: [64.0 ("Value") 0.5 ("Value") 1.0 ("Value")] -> w243
              frame "PWM" {
              }
              frame "Motor", Default {
              }
              frame "Analog Out" {
              }
            }
            n136 = property on="Motor" class="Clust (strict)"("Visible"=TRUE) -> ()  [unwired: 2 in, 2 out]
            n137 = property on="Value" class="Slide (strict)"("Value"=w244, "Scale.Minimum"=w246, "Scale.Maximum"=w245, "Scale.Increment"=w243) -> ()  [unwired: 2 in, 2 out]
            n138 = property on="On/Off" class="Bool (strict)"("Visible"=w248) -> ()  [unwired: 2 in, 2 out]
            n139 = property on="Test Slider" class="Slide (strict)"("Visible"=w248) -> ()  [unwired: 2 in, 2 out]
            n140 = property on="Test Ring" class="Ring (strict)"("Visible"=w248) -> ()  [unwired: 2 in, 2 out]
            n141 = property on="Rev/Fwd" class="Clust (strict)"("Visible"=w248) -> ()  [unwired: 2 in, 2 out]
          }
          frame "Servo" {
            w264 = FALSE ("Visible")
            n142 = call <vilib>:"NT Read Number.vi"("Name"=w266) -> ("Numeric"=w265:dbl)  [unwired: 9 in, 1 out]
            n143 = property on="Test Slider" class="Slide (strict)"("Visible"=TRUE, "Scale.Maximum"=170.0 ("Scale.Range:Maximum")) -> ()  [unwired: 2 in, 2 out]
            n144 = local write "Test Slider"(w265) -> ()
            n145 = property on="Motor" class="Clust (strict)"("Visible"=w264) -> ()  [unwired: 2 in, 2 out]
            n146 = property on="Rev/Fwd" class="Clust (strict)"("Visible"=w264) -> ()  [unwired: 2 in, 2 out]
            n147 = property on="On/Off" class="Bool (strict)"("Visible"=w264) -> ()  [unwired: 2 in, 2 out]
            n148 = property on="Test Ring" class="Ring (strict)"("Visible"=w264) -> ()  [unwired: 2 in, 2 out]
          }
          frame "Relay", "Solenoid" {
            w267 = FALSE ("Visible")
            n149 = property on="Motor" class="Clust (strict)"("Visible"=w267) -> ()  [unwired: 2 in, 2 out]
            n150 = property on="Test Slider" class="Slide (strict)"("Visible"=w267) -> ()  [unwired: 2 in, 2 out]
            n151 = Search and Replace String(input string=w268, search string="/Value  **", replace string="/Direction") -> (result string=w274:string)  [unwired: 5 in, 3 out]
            n152 = property on="Test Ring" class="Ring (strict)"("Visible"=w267) -> ()  [unwired: 2 in, 2 out]
            n153 = call <vilib>:"NT Read String.vi"("Name"=w274) -> ("String"=w272:string)  [unwired: 9 in, 1 out]
            n154 = Equal?(x="Both directions", y=w272) -> (x = y?=w270:bool)
            n155 = Not(x=w270) -> (.not. x?=w271:bool)
            n156 = property on="Rev/Fwd" class="Clust (strict)"("Visible"=w270) -> ()  [unwired: 2 in, 2 out]
            n157 = property on="On/Off" class="Bool (strict)"("Visible"=w271, "Caption.Text"=w269) -> ()  [unwired: 2 in, 2 out]
          }
          frame "Compressor", "Digital Out" {
            w277 = FALSE ("Visible")
            # "Get direction and finish"
            n158 = property on="Motor" class="Clust (strict)"("Visible"=w277) -> ()  [unwired: 2 in, 2 out]
            n159 = property on="Test Slider" class="Slide (strict)"("Visible"=w277) -> ()  [unwired: 2 in, 2 out]
            n160 = property on="Test Ring" class="Ring (strict)"("Visible"=w277) -> ()  [unwired: 2 in, 2 out]
            n161 = property on="On/Off" class="Bool (strict)"("Visible"=TRUE, "Caption.Text"=w278) -> ()  [unwired: 2 in, 2 out]
            n162 = property on="Rev/Fwd" class="Clust (strict)"("Visible"=FALSE) -> ()  [unwired: 2 in, 2 out]
          }
          frame "Camera" {
            n163 = call <vilib>:"Get Last Path Segment.vi"("String in"=w285) -> ("String out"=w286:string)  [unwired: 10 in]
            n164 = property on="On/Off" class="Bool (strict)"("Visible"=FALSE) -> ()  [unwired: 2 in, 2 out]
            n165 = property on="Motor" class="Clust (strict)"("Visible"=FALSE) -> ()  [unwired: 2 in, 2 out]
            n166 = property on="Rev/Fwd" class="Clust (strict)"("Visible"=FALSE) -> ()  [unwired: 2 in, 2 out]
            n167 = case shown="\"White Balance  **\"" w286 {
              tunnel: w285 -> [w292 w301 w310 w319 w328 _ w334]
              tunnel: w284 -> [w290 w298 w307 w316 w325 _ _]
              frame "Size  **" {
                n168 = Index Array(array=w290) -> (element=w289:cluster{string[]})  [unwired: 1 in]
                n169 = call <vilib>:"NT Read String.vi"("Name"=w292) -> ("String"=w291:string)  [unwired: 9 in, 1 out]
                n170 = Unbundle(w289) -> (w287:string[])
                n171 = Match First String(2:w287, 3:w291) -> (0:w288:i32)  [unwired: 1 out]
                n172 = property on="Test Ring" class="Ring (strict)"("Value"=w288, "Strings []"=w287) -> ()  [unwired: 2 in, 2 out]
                n173 = property on="Test Ring" class="Ring (strict)"("Visible"=TRUE) -> ()  [unwired: 2 in, 2 out]
                n174 = property on="Test Slider" class="Slide (strict)"("Visible"=FALSE) -> ()  [unwired: 2 in, 2 out]
              }
              frame "White Balance  **" {
                n175 = Index Array(array=w298, index=1) -> (element=w299:cluster{string[]})
                n176 = call <vilib>:"NT Read String.vi"("Name"=w301) -> ("String"=w300:string)  [unwired: 9 in, 1 out]
                n177 = Unbundle(w299) -> (w296:string[])
                n178 = Match First String(2:w296, 3:w300) -> (0:w295:i32)  [unwired: 1 out]
                n179 = property on="Test Ring" class="Ring (strict)"("Value"=w295, "Strings []"=w296) -> ()  [unwired: 2 in, 2 out]
                n180 = property on="Test Ring" class="Ring (strict)"("Visible"=TRUE) -> ()  [unwired: 2 in, 2 out]
                n181 = property on="Test Slider" class="Slide (strict)"("Visible"=FALSE) -> ()  [unwired: 2 in, 2 out]
              }
              frame "Exposure  **" {
                n182 = Index Array(array=w307, index=2) -> (element=w308:cluster{string[]})
                n183 = call <vilib>:"NT Read String.vi"("Name"=w310) -> ("String"=w309:string)  [unwired: 9 in, 1 out]
                n184 = Unbundle(w308) -> (w304:string[])
                n185 = Match First String(2:w304, 3:w309) -> (0:w305:i32)  [unwired: 1 out]
                n186 = property on="Test Ring" class="Ring (strict)"("Value"=w305, "Strings []"=w304) -> ()  [unwired: 2 in, 2 out]
                n187 = property on="Test Ring" class="Ring (strict)"("Visible"=TRUE) -> ()  [unwired: 2 in, 2 out]
                n188 = property on="Test Slider" class="Slide (strict)"("Visible"=FALSE) -> ()  [unwired: 2 in, 2 out]
              }
              frame "Exposure Priority  **" {
                n189 = Index Array(array=w316, index=3) -> (element=w317:cluster{string[]})
                n190 = call <vilib>:"NT Read String.vi"("Name"=w319) -> ("String"=w318:string)  [unwired: 9 in, 1 out]
                n191 = Unbundle(w317) -> (w313:string[])
                n192 = Match First String(2:w313, 3:w318) -> (0:w314:i32)  [unwired: 1 out]
                n193 = property on="Test Ring" class="Ring (strict)"("Value"=w314, "Strings []"=w313) -> ()  [unwired: 2 in, 2 out]
                n194 = property on="Test Ring" class="Ring (strict)"("Visible"=TRUE) -> ()  [unwired: 2 in, 2 out]
                n195 = property on="Test Slider" class="Slide (strict)"("Visible"=FALSE) -> ()  [unwired: 2 in, 2 out]
              }
              frame "Color Enable  **" {
                n196 = Index Array(array=w325, index=4) -> (element=w326:cluster{string[]})
                n197 = call <vilib>:"NT Read String.vi"("Name"=w328) -> ("String"=w327:string)  [unwired: 9 in, 1 out]
                n198 = Unbundle(w326) -> (w322:string[])
                n199 = Match First String(2:w322, 3:w327) -> (0:w323:i32)  [unwired: 1 out]
                n200 = property on="Test Ring" class="Ring (strict)"("Value"=w323, "Strings []"=w322) -> ()  [unwired: 2 in, 2 out]
                n201 = property on="Test Ring" class="Ring (strict)"("Visible"=TRUE) -> ()  [unwired: 2 in, 2 out]
                n202 = property on="Test Slider" class="Slide (strict)"("Visible"=FALSE) -> ()  [unwired: 2 in, 2 out]
              }
              frame Default {
                n203 = property on="Test Ring" class="Ring (strict)"("Visible"=FALSE) -> ()  [unwired: 2 in, 2 out]
                n204 = property on="Test Slider" class="Slide (strict)"("Visible"=FALSE) -> ()  [unwired: 2 in, 2 out]
              }
              frame "Brightness  **", "Color Level  **", "Compression  **", "FPS  **", "Sharpness  **" {
                n205 = call <vilib>:"NT Read Number.vi"("Name"=w334) -> ("Numeric"=w333:dbl)  [unwired: 9 in, 1 out]
                n206 = local write "Test Slider"(w333) -> ()
                n207 = property on="Test Slider" class="Slide (strict)"("Visible"=TRUE, "Scale.Maximum"=100.0 ("Scale.Range:Maximum")) -> ()  [unwired: 2 in, 2 out]
                n208 = property on="Test Ring" class="Ring (strict)"("Visible"=FALSE) -> ()  [unwired: 2 in, 2 out]
              }
            }
          }
        }
        n209 = property on="Progress" class="Clust (strict)"("Visible"=FALSE) -> ()  [unwired: 2 in, 2 out]
      }
      event "Test Name": Mouse Enter {
        # "Populate the ring with the list of tests"
        n210 = event-data() -> ()  [unwired: 1 in, 1 out]
        n211 = call <vilib>:"NT Read String Array.vi"("Name"="TestMode/TestList") -> ("String Array"=w342:string[])  [unwired: 9 in, 1 out]
        n212 = Build Array (concatenate)("Select the test to run...", w342) -> (w341:string[])
        n213 = property on="Test Name" class="Ring (strict)"("Strings []"=w341) -> ()  [unwired: 2 in, 2 out]
      }
      event "Test Name": Value Change {
        w344 = FALSE ("Visible")
        # "Tell the robot the test name to run"
        n214 = event-data() -> ("NewVal"=w348:u16)  [unwired: 1 in]
        n215 = property on="Test Name" class="Ring (strict)"() -> ("Strings []"=w349:string[])  [unwired: 2 in, 2 out]
        n216 = local write "Progress"(T6 {"Test Progress"=0, "Test Progress Text"=""} ("Progress")) -> ()
        n217 = Index Array(array=w349, index=w348) -> (element=w347:string)
        n218 = call <vilib>:"NT Write String.vi"("String"=w347, "Name"="TestMode/TestName") -> ()  [unwired: 9 in, 1 out]
        n219 = property on="Progress" class="Clust (strict)"("Visible"=TRUE) -> ()  [unwired: 2 in, 2 out]
        n220 = property on="Motor" class="Clust (strict)"("Visible"=w344) -> ()  [unwired: 2 in, 2 out]
        n221 = property on="Test Slider" class="Slide (strict)"("Visible"=w344) -> ()  [unwired: 2 in, 2 out]
        n222 = property on="On/Off" class="Bool (strict)"("Visible"=w344) -> ()  [unwired: 2 in, 2 out]
        n223 = property on="Rev/Fwd" class="Clust (strict)"("Visible"=w344) -> ()  [unwired: 2 in, 2 out]
        n224 = property on="Test Ring" class="Ring (strict)"("Visible"=w344) -> ()  [unwired: 2 in, 2 out]
      }
      event "Select Auto": Mouse Enter {
        # "Populate the combo box with the list of autonomous options"
        n225 = event-data() -> ()  [unwired: 1 in, 1 out]
        n226 = call <vilib>:"NT Read String Array.vi"("Name"="Auto List") -> ("String Array"=w351:string[])  [unwired: 9 in, 1 out]
        n227 = property on="Select Auto" class="CmbBox"("Strings[]"=w351) -> ()  [unwired: 2 in, 2 out]
      }
      event "Select Pickup": Mouse Enter {
        n228 = event-data() -> ()  [unwired: 1 in, 4 out]
        n229 = call <vilib>:"NT Read String Array.vi"("Name"="Auto Pickup") -> ("String Array"=w354:string[])  [unwired: 9 in, 1 out]
        n230 = property on="Select Pickup" class="CmbBox"("Strings[]"=w354) -> ()  [unwired: 2 in, 2 out]
      }
      event "Select Auto": Value Change {
        # "User modified the Auto Selection. Write to NT variable so robot knows."
        n231 = event-data() -> ("NewVal"=w357:string)  [unwired: 1 in]
        n232 = call <vilib>:"NT Write String.vi"("String"=w357, "Name"="Auto Selector") -> ()  [unwired: 9 in, 1 out]
      }
      event "Select Pickup": Value Change {
        # "User modified the Auto Selection. Write to NT variable so robot knows."
        n233 = event-data() -> ("NewVal"=w360:string)  [unwired: 1 in]
        n234 = call <vilib>:"NT Write String.vi"("String"=w360, "Name"="Auto Pickup Selector") -> ()  [unwired: 9 in, 1 out]
      }
      event "Command Selection": Value Change {
        # "Get the params and show in table"
        n235 = event-data() -> ("NewVal"=w366:i32)  [unwired: 1 in]
        n236 = property on="Command Selection" class="MCListbox (strict)"() -> ("ItemNames"=w364:string[][])  [unwired: 2 in, 2 out]
        n237 = call <vilib>:"WPI_DashboardUpdate Command Params.vi"("NewVal"=w366, "Commands"=w364, "Param Tbl"=w365) -> ()  [unwired: 8 in, 1 out]
      }
      event "Execute Command": Value Change {
        # "Started one, Unique ID holds\nresponse"
        n238 = event-data() -> ()  [unwired: 1 in, 1 out]
        n239 = property on="Command Selection" class="MCListbox (strict)"() -> ("ItemNames"=w377:string[][])  [unwired: 2 in, 2 out]
        n240 = Index Array(array=w377, index (row)="Command Selection", index (col)=0) -> (element=w375:string)
        n241 = call <vilib>:"Invoke Commands.vi"("Command Params"="Command Params", "Function Name"=w375) -> ("Params"=w371:u8, "Started"=w370:bool)  [unwired: 7 in, 1 out]
        n242 = Array Subset(array="Command Params", length (row)=w371) -> (w372:string[][])  [unwired: 3 in]
        n243 = Select(t="Executing" ("Cmd Status"), s=w370, f="" ("Cmd Status")) -> (s? t:f=→"Cmd Status":string)
      }
      event "Command Selection": Double Click {
        n244 = event-data() -> ("Row"=w385:i32)  [unwired: 1 in]
        n245 = property on="Command Selection" class="MCListbox (strict)"() -> ("ItemNames"=w388:string[][])  [unwired: 2 in, 2 out]
        n246 = local read "Command Params"() -> (w384:string[][])
        n247 = Index Array(array=w388, index (row)=w385, index (col)=0) -> (element=w386:string)
        n248 = call <vilib>:"Invoke Commands.vi"("Command Params"=w384, "Function Name"=w386) -> ("Params"=w383:u8, "Started"=w378:bool)  [unwired: 7 in, 1 out]
        n249 = Array Subset(array=w384, length (row)=w383) -> (w382:string[][])  [unwired: 3 in]
        n250 = Select(t="Executing" ("Cmd Status"), s=w378, f="" ("Cmd Status")) -> (s? t:f=w379:string)
        n251 = local write "Cmd Status"(w379) -> ()
      }
      event "CheckList": Double Click {
        # "Shift clears all"
        # "Update symbols on the listbox"
        n252 = event-data() -> ("PlatMods.Shift"=w390:bool, "Row"=w392:i32)  [unwired: 1 in]
        n253 = case shown="True" w390 {
          tunnel: w392 -> [w396 _]
          tunnel: 1 -> [w395 _]
          frame False {
            n254 = property on="CheckList" class="LstBox (strict)"() -> ("Item Symbols"=w394:i32[])  [unwired: 2 in, 2 out]
            n255 = Replace Array Subset(array=w394, new element=w395, index=w396) -> (w393:i32[])
            n256 = property on="CheckList" class="LstBox (strict)"("Item Symbols"=w393) -> ()  [unwired: 2 in, 2 out]
          }
          frame True {
            w397 = 0 ("Top Row")
            n257 = property on="CheckList" class="LstBox (strict)"() -> ("Number of Rows"=w399:u32)  [unwired: 2 in, 2 out]
            n258 = Initialize Array(0, w399) -> (w398:i32[])
            n259 = property on="CheckList" class="LstBox (strict)"("Top Row"=w397, "Value"=w397, "Item Symbols"=w398) -> ()  [unwired: 2 in, 2 out]
          }
        }
      }
      event "CheckList": Key Down {
        # "Update symbols on the listbox\nLeft and right keys check and uncheck"
        n260 = event-data() -> ("VKey"=w403:T22)  [unwired: 1 in]
        n261 = case shown="\"Left\", \"Right\"" w403 {
          selector: w403 -> [w408 _]
          tunnel: eventvkey."Left" ("VKey") -> [w406 _]
          frame "Left", "Right" {
            n262 = Equal?(x=w406, y=w408) -> (x = y?=w407:bool)
            n263 = Select(t=0, s=w407, f=1) -> (s? t:f=w409:i32)
            n264 = property on="CheckList" class="LstBox (strict)"() -> ("Item Symbols"=w412:i32[])  [unwired: 2 in, 2 out]
            n265 = Replace Array Subset(array=w412, new element=w409, index="CheckList") -> (w411:i32[])
            n266 = property on="CheckList" class="LstBox (strict)"("Item Symbols"=w411) -> ()  [unwired: 2 in, 2 out]
          }
          frame Default {
          }
        }
      }
      event "Motor.Enable": Value Change {
        # "When the test mode otor enable helper is set, update that\ntree row item's value"
        n267 = event-data() -> ("NewVal"=w418:bool)  [unwired: 1 in]
        n268 = Unbundle("Motor") -> ("Value"=w417:dbl)  [unwired: 1 out]
        n269 = Select(t=w417, s=w418, f=0.0) -> (s? t:f=w415:dbl)
        n270 = call <vilib>:"NT Write Number.vi"("Numeric"=w415, "Name"=w414) -> ()  [unwired: 9 in, 1 out]
      }
      event "Test Slider": Value Change {
        # "When the test mode slider helper is set, update that\ntree row item's value"
        n271 = event-data() -> ("NewVal"=w421:dbl)  [unwired: 1 in]
        n272 = call <vilib>:"NT Write Number.vi"("Numeric"=w421, "Name"=w422) -> ()  [unwired: 9 in, 1 out]
      }
      event "On/Off": Value Change {
        # "When the test mode on/off helper value is set, update that\ntree row item's value"
        n273 = event-data() -> ("NewVal"=w426:bool)  [unwired: 1 in]
        n274 = Boolean To (0,1)(Boolean=w426) -> (0, 1=w425:i16)
        n275 = call <vilib>:"NT Write Number.vi"("Numeric"=w425, "Name"=w424) -> ()  [unwired: 9 in, 1 out]
      }
      event "Rev/Fwd": Value Change {
        # "When the test mode helper value for relays is set, update that\ntree row item's value"
        n276 = event-data() -> ("NewVal.Forward"=w434:bool, "NewVal.Reverse"=w433:bool)  [unwired: 1 in]
        n277 = Boolean To (0,1)(Boolean=w434) -> (0, 1=w430:i16)
        n278 = Boolean To (0,1)(Boolean=w433) -> (0, 1=w432:i16)
        n279 = Negate(x=w432) -> (-x=w431:i16)
        n280 = Add(x=w430, y=w431) -> (x+y=w429:i16)
        n281 = call <vilib>:"NT Write Number.vi"("Numeric"=w429, "Name"=w428) -> ()  [unwired: 9 in, 1 out]
      }
      event "Test Ring": Value Change {
        # "When a test mode helper value is selected from the ring,\nset the tree item's variable to the string value"
        n282 = event-data() -> ("NewVal"=w438:u16)  [unwired: 1 in]
        n283 = property on="Test Ring" class="Ring (strict)"() -> ("Strings []"=w439:string[])  [unwired: 2 in, 2 out]
        n284 = Index Array(array=w439, index=w438) -> (element=w437:string)
        n285 = call <vilib>:"NT Write String.vi"("String"=w437, "Name"=w436) -> ()  [unwired: 9 in, 1 out]
      }
      event "Rec Mode": Value Change {
        # "Update globals for recording mode and path to read log from.\nClear when logging and let NetworkTables set path for vision to\nuse."
        n286 = event-data() -> ("NewVal"=w450:enum32{"Stop", "Record", "Playback"})  [unwired: 1 in]
        n287 = global write "WPI_DashboardLogging Global.vi" "Logging Filename"(path "") -> ()
        n288 = global write "WPI_DashboardLogging Global.vi" "Recording"(w450) -> ()
        n289 = case shown="\"Playback\"" w450 {
          tunnel: w449 -> [_ w452 w461]
          tunnel: [_ _ w460] -> w447
          tunnel: [_ _ w459] -> _
          tunnel: w445 -> [_ _ w457]
          tunnel: cluster{i32, i32} {-250, 170} -> [_ _ w456]
          tunnel: [_ _ T23 {"Image Size"=TRUE, "Image Type"=TRUE, "Pixel Value"=TRUE, "ROI Information"=TRUE, "Zoom Factor"=FALSE} ("Image Information Shown:All Elements")] -> w440
          tunnel: [_ _ TRUE ("Zoom Factor")] -> w441
          tunnel: w443 -> [_ _ w453]
          frame Default {
          }
          frame "Stop", "Record" {
            # "Place Window too"
            n290 = invoke class="VI" method="FP.Close"(reference=w452) -> (reference out=w451:refnum<vi>)  [unwired: 2 in, 2 out]
            n291 = invoke class="VI" method="Abort VI"(reference=w451) -> ()  [unwired: 2 in, 3 out]
          }
          frame "Playback" {
            n292 = call "Open Playback Panel.vi"("Offset"=w456, "DB VI Ref"=w457, "Playback in"=w461) -> ("Playback out"=w458:refnum<vi>)  [unwired: 8 in]
            n293 = register-events(w458, w453) -> (reference out=w460:refnum<event-registration>, error out=w459:errorcluster)  [unwired: 2 in]
          }
        }
        n294 = property on="Camera Image Right" class="ImageControl"("Image Information Shown"=w440, "Image Information Visible"=w441) -> ()  [unwired: 2 in, 2 out]
        n295 = property on="Camera Image" class="ImageControl"("Image Information Shown"=w440, "Image Information Visible"=w441) -> ()  [unwired: 2 in, 2 out]
        n296 = call <vilib>:"WPI_DashboardNT Log FieldName Cache.vi"("Operation"=enum16{"Lookup/Add", "Index", "Clear"}."Clear") -> ()  [unwired: 8 in, 3 out]
      }
      event Panel Close {
        w463 = enum32{"Stop", "Record", "Playback"}."Stop" ("Rec Mode")
        # "Playback window has been closed, abort"
        n297 = event-data() -> ()  [unwired: 1 in, 4 out]
        n298 = local write "Rec Mode"(w463) -> ()
        n299 = global write "WPI_DashboardLogging Global.vi" "Recording"(w463) -> ()
      }
      event Panel Close {
        # "Abort playback window and ourself"
        n300 = event-data() -> ()  [unwired: 1 in, 4 out]
        n301 = invoke class="VI" method="FP.Close"(reference=w467) -> (reference out=w466:refnum<vi>)  [unwired: 2 in, 2 out]
        n302 = invoke class="VI" method="Abort VI"(reference=w466) -> (error out=w465:errorcluster)  [unwired: 2 in, 2 out]
        n303 = invoke class="VI" method="Abort VI"(error in=w465) -> ()  [unwired: 2 in, 3 out]
      }
      event User Event {
        n304 = event-data() -> ("IDs"=w474:cluster{"RPC field ID":u16, "Unique ID":u16}, "String"=w473:string)  [unwired: 1 in]
        n305 = Bundle("IDs"=w474, "String"=w473) -> (w472:T9)  [unwired: 1 in]
        n306 = call <vilib>:"Retrieve RPC Response.vi"("RPC Response"=w472) -> ("Output"=w470:string[][])  [unwired: 10 in]
        n307 = Build Array (concatenate)(w468, w470) -> (w469:string[][])
        n308 = local write "Command Params"(w469) -> ()
        n309 = local write "Cmd Status"("" ("Cmd Status")) -> ()
      }
      event "Tree": Double Click {
        n310 = event-data() -> ("PlatMods"=w480:T26, "Tag"=w477:string)  [unwired: 1 in]
        n311 = Unbundle(w480) -> ("Shift"=w479:bool)  [unwired: 4 out]
        n312 = String Subset(string=w477, length (rest)=1 ("length (rest)")) -> (substring=w476:string)  [unwired: 1 in]
        n313 = Not(x=w479) -> (.not. x?=w478:bool)
        n314 = case shown="\"/\"" w476 {
          tunnel: w477 -> [_ w483]
          tunnel: w478 -> [_ w482]
          frame Default {
          }
          frame "/" {
            n315 = call <vilib>:"NT Update Persistence.vi"("Persistence"=w482, "Name"=w483) -> ()  [unwired: 9 in, 1 out]
          }
        }
      }
    }
  }
  n316 = while {
    tunnel: w67 -> [w485]
    i -> [w488]
    stop <- FALSE stop-if-true
    n317 = Wait (ms)(milliseconds to wait=u32 100) -> ()  [unwired: 1 out]
    n318 = case shown="\"Playback\"" "Rec Mode" {
      tunnel: w488 -> [_ _ w503]
      tunnel: [u32 2829099 ("Base Color") u32 11141120 ("Target Color") w492] -> w484
      frame "Stop", Default {
        # "Reset the color, extra updates don't cost much"
      }
      frame "Record" {
      }
      frame "Playback" {
        # "Playback"
        n319 = Quotient & Remainder(x=w503, y=u32 50 ("milliseconds to wait")) -> (x-y*floor(x/y)=w499:u32)  [unwired: 1 out]
        n320 = Divide(x=w499, y=u32 50 ("milliseconds to wait")) -> (x/y=w496:dbl)
        n321 = Multiply(x=6.283185307179586, y=w496) -> (x*y=w501:dbl)
        n322 = Sine(x=w501) -> (sin(x)=w500:dbl)
        n323 = Absolute Value(x=w500) -> (abs(x)=w493:dbl)
        n324 = call "Interpolate RGB Color.vi"("Proportion"=w493, "Target Color"=u32 30976, "Base Color"=u32 2829099) -> ("Result Color"=w492:u32)  [unwired: 8 in]
      }
    }
    n325 = property class="Pane"(reference=w485, "PaneColor"=w484) -> ()  [unwired: 1 in, 2 out]
  }
  n326 = local write "Dashboard Tab"(T2."Drive" ("Dashboard Tab")) -> ()
  n327 = property on="On/Off" class="Bool (strict)"("Visible"=w38) -> ()  [unwired: 2 in, 2 out]
  n328 = property on="Motor" class="Clust (strict)"("Visible"=w38) -> ()  [unwired: 2 in, 2 out]
  n329 = property on="Progress" class="Clust (strict)"("Visible"=w38) -> ()  [unwired: 2 in, 2 out]
  n330 = property on="Test Ring" class="Ring (strict)"("Visible"=w38) -> ()  [unwired: 2 in, 2 out]
  n331 = property on="Rev/Fwd" class="Clust (strict)"("Visible"=w38) -> ()  [unwired: 2 in, 2 out]
  n332 = while {
    tunnel: u16 1741 ("timeout ms (25000)") -> [w505]
    stop <- FALSE stop-if-true
    n333 = TCP Create Listener(10:w505) -> (0:w504:errorcluster, 3:w506:refnum<k5>)  [unwired: 4 in, 1 out]
    n334 = case shown="No Error" w504 {
      selector: w504 -> [w508 _]
      tunnel: w506 -> [w509 _]
      frame No Error {
        n335 = while {
          tunnel: w509 -> [w512]
          tunnel: w508 -> [w511]
          stop <- FALSE stop-if-true
          n336 = TCP Wait On Listener(8:w511, 11:w512) -> (0:w513:errorcluster, 4:w514:refnum<k5>)  [unwired: 2 in, 3 out]
          n337 = local write "TCP"(w514) -> ()
          n338 = case shown="No Error" w513 {
            frame No Error {
            }
            frame Error {
              n339 = Wait (ms)(milliseconds to wait=u32 1000) -> ()  [unwired: 1 out]
            }
          }
        }
      }
      frame Error {
        n340 = Wait (ms)(milliseconds to wait=u32 1000) -> ()  [unwired: 1 out]
      }
    }
  }
  n341 = local write "Command Selection"(u16 0 ("milliseconds to wait")) -> ()
  n342 = local write "Command Params"(string[][] [] ("Command Params")) -> ()
  n343 = call <vilib>:"NT Write String.vi"("String"="Select Auto", "Name"="Auto Selector") -> ()  [unwired: 9 in, 1 out]
  n344 = global write "WPI_DashboardLogging Global.vi" "Recording"(w61) -> ()
  n345 = local write "Rec Mode"(w61) -> ()
  n346 = call <vilib>:"NT Write String.vi"("String"="Select Pickup", "Name"="Auto Pickup Selector") -> ()  [unwired: 9 in, 1 out]
